vi "TDT-Stop.vi"(11 "error in (no error)":errorcluster) -> (15 "error out":errorcluster)   [LabVIEW 2020]
doc: "Sets global variables that terminate the main DAQ loop."
uses:
  TDT-Globals.vi
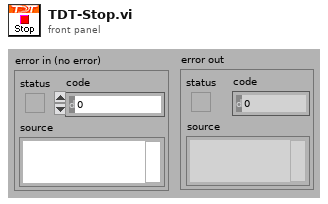
[diagram p1: front panel]
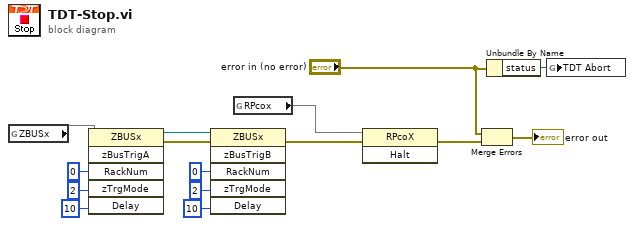
[diagram p0: block diagram]
diagram:
  n1 = global read "TDT-Globals.vi" "ZBUSx"() -> (w1)
  n2 = invoke class="ZBUSx" method="zBusTrigA"(reference=w1, "RackNum"=0, "zTrgMode"=2, "Delay"=10) -> (reference out=w5:refnum<k7>, error out=w4:errorcluster)  [unwired: 2 in, 4 out]
  n3 = invoke class="ZBUSx" method="zBusTrigB"(reference=w5, error in=w4, "RackNum"=0, "zTrgMode"=2, "Delay"=10) -> (error out=w3:errorcluster)  [unwired: 1 in, 5 out]
  n4 = global read "TDT-Globals.vi" "RPcox"() -> (w2)
  n5 = invoke class="RPcoX" method="Halt"(reference=w2, error in=w3) -> (error out=w12:errorcluster)  [unwired: 1 in, 2 out]
  n6 = Merge Errors("error in (no error)", w12) -> (→"error out":errorcluster)
  n7 = Unbundle By Name("error in (no error)") -> ("status"=w9:bool)
  n8 = global write "TDT-Globals.vi" "TDT Abort"(w9) -> ()
